vi "Measurement Logic.vi"(8 "error in":errorcluster, 10 "Measurement Context":refnum<class "MeasurementContext.lvclass">, 11 "Measurement Configuration":T2) -> (0 "error out":errorcluster, 2 "Measurement Context out":refnum<class "MeasurementContext.lvclass">, 3 "Measurement Results":T1 {"Load Regulation (mV/mA)" format="%#.5g"})   [LabVIEW 2020, in "LoadRegulation.lvlib"]
uses:
  LoadRegulation.lvlib
  Measurement Configuration.ctl
  Measurement Results.ctl
  RPC Service/MeasurementContext/MeasurementContext.lvclass
  TestInputs.ctl
  Reusables/Advanced Settings.ctl
  Reusables/Prepare Fn Configurations.ctl
  Reusables/Load Output Function.ctl
  Reusables/Stimulus And Measure.ctl
  TestResults.ctl
  e7ccc9a1-0b5d-4153-a5a6-c1ed66e62fb2.vi
panel:
  out "Load Regulation":cluster{"Iload (mA)":dbl[], "Vout (V)":dbl[]}(graph)
  out "Load Regulation (%)":dbl format="%#.3g"
  out "Load Regulation (mV/mA)":dbl format="%#.3g"
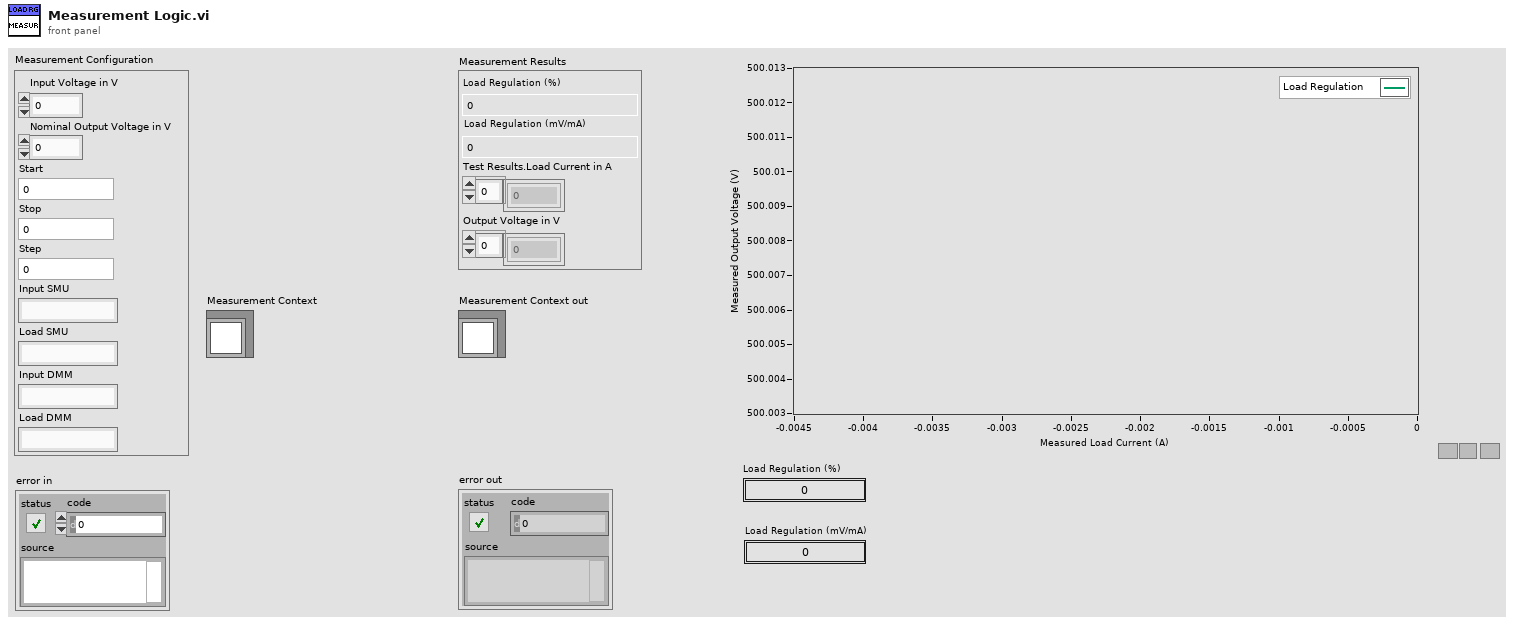
[diagram p1: front panel]
types:
  T1 = typedef "LoadRegulation.lvlib/Measurement Results.ctl" = cluster{"Load Regulation (%)":dbl, "Load Regulation (mV/mA)":dbl, "Test Results.Load Current in A":dbl[], "Output Voltage in V":dbl[]}
  T2 = typedef "LoadRegulation.lvlib/Measurement Configuration.ctl" = cluster{"Input Voltage in V":dbl, "Nominal Output Voltage in V":dbl, "Start":dbl, "Stop":dbl, "Step":dbl, "Input SMU":string, "Load SMU":string, "Input DMM":string, "Load DMM":string}
  T3 = typedef "LoadRegulation.lvlib/TestInputs.ctl" = cluster{"Input Voltage in V":dbl, "Load Current in A":dbl[], "Nominal Output Voltage in V":dbl, "Advance Setting":T4}
  T4 = typedef "Advanced Settings.ctl" = cluster{"Prepare":T5, "Stimulus And Measure":T7}
  T5 = typedef "Prepare Fn Configurations.ctl" = cluster{"Load SMU Output Function":T6}
  T6 = typedef "Load Output Function.ctl" = enum16{"VoltageSource", "CurrentSource"}
  T7 = typedef "Stimulus And Measure.ctl" = cluster{"Loop Delay in milliSecond":u32}
  T8 = typedef "LoadRegulation.lvlib/TestResults.ctl" = cluster{"Input Voltage in V":dbl[], "Input Current in A":dbl[], "Output Voltage in V":dbl[], "Load Current in A":dbl[], "Load Regulation in mV/mA":dbl, "Load Regulation in %":dbl}
  T9 = cluster{"Test Inputs":T3, "Test Results":T8, "Test Results[][]":string[][], "Input SMU":refnum<k15>, "Input DMM":refnum<k15>, "Load DMM":refnum<k15>, "Load SMU":refnum<k15>}
  T10 = cluster{"Load Current in A":dbl[], "Output Voltage in V":dbl[]}
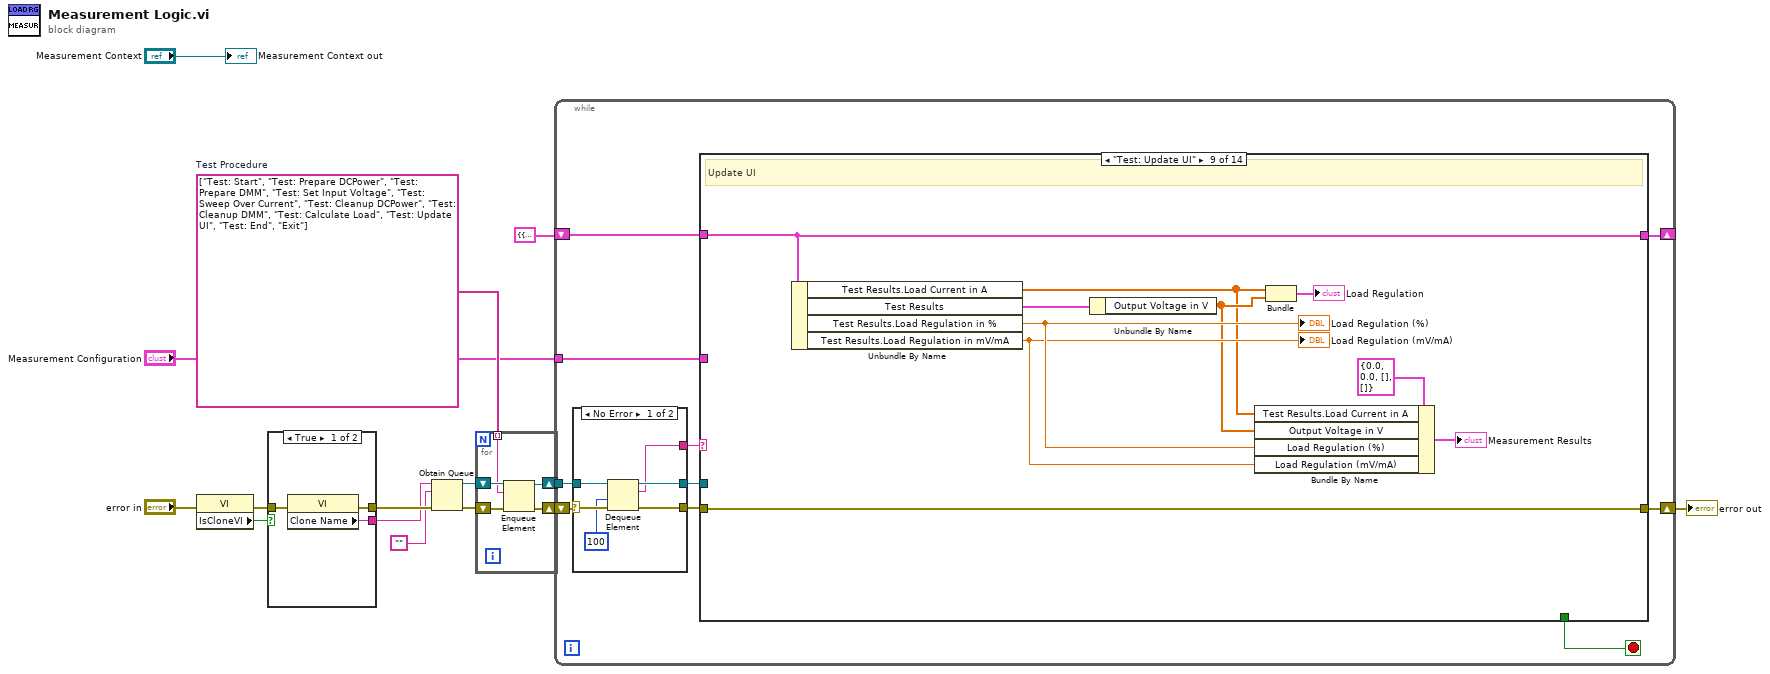
[diagram p0: block diagram]
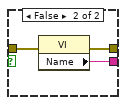
[diagram p2: hidden frame]
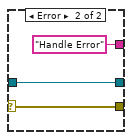
[diagram p3: hidden frame]
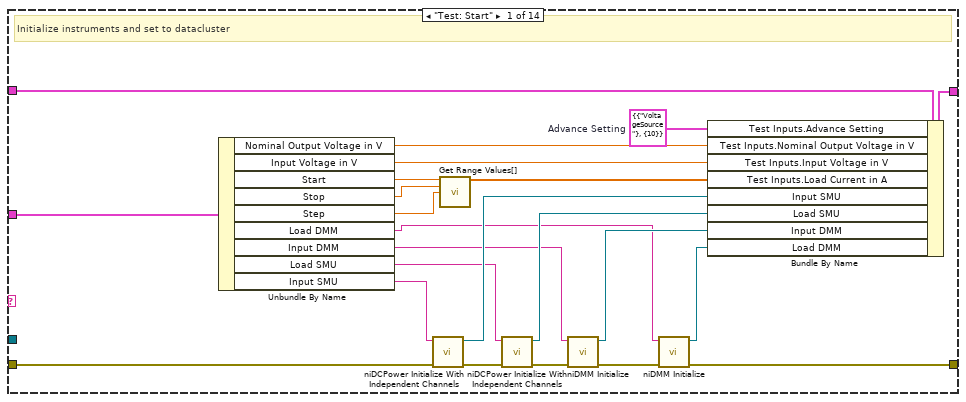
[diagram p4: hidden frame]
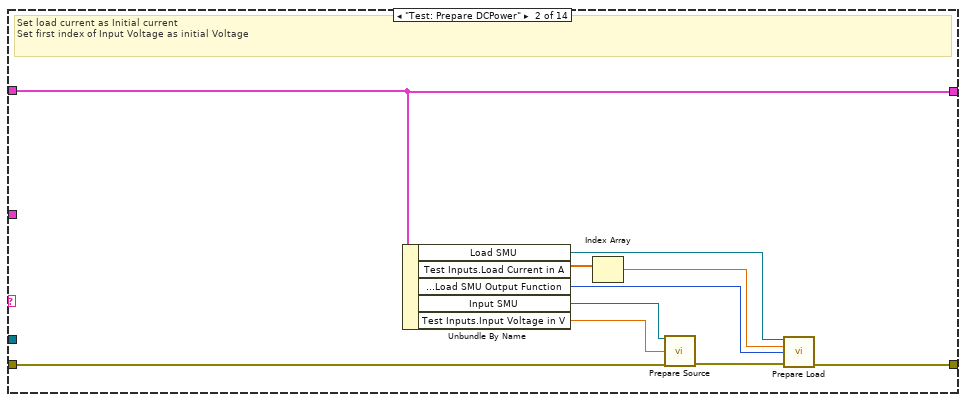
[diagram p5: hidden frame]
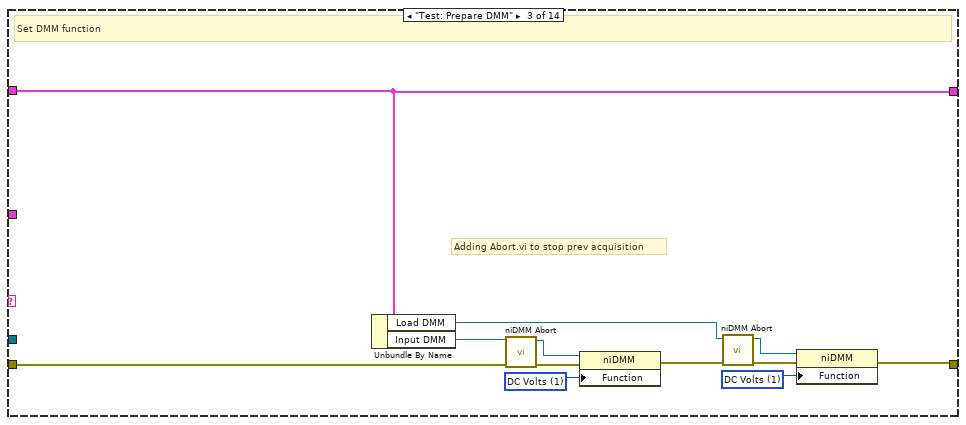
[diagram p6: hidden frame]
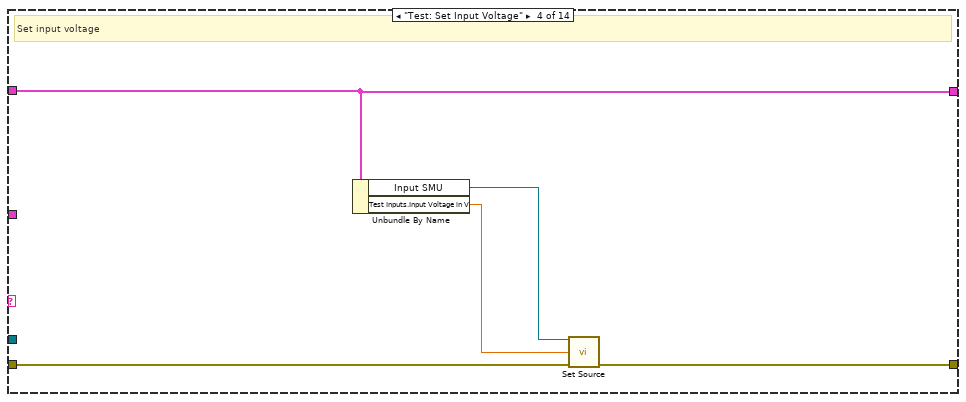
[diagram p7: hidden frame]
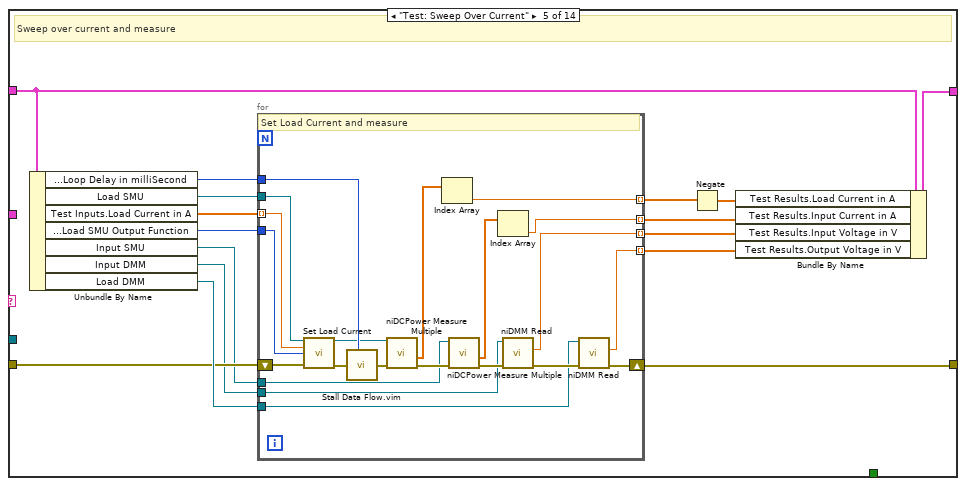
[diagram p8: hidden frame]
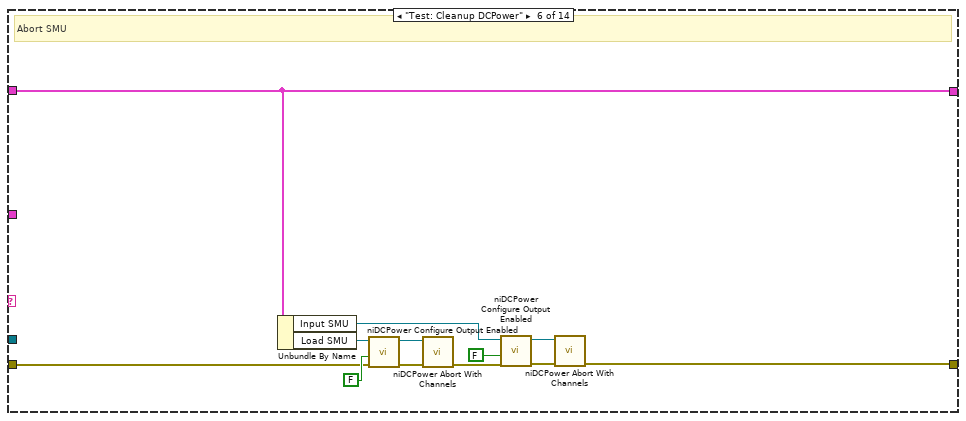
[diagram p9: hidden frame]
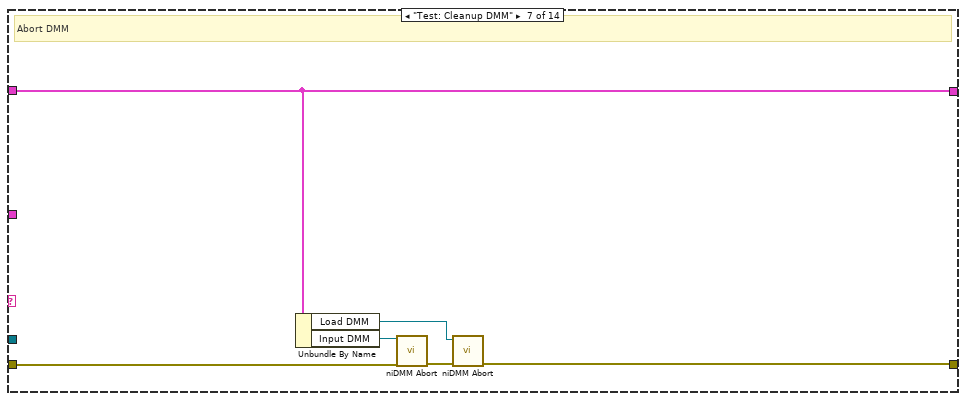
[diagram p10: hidden frame]
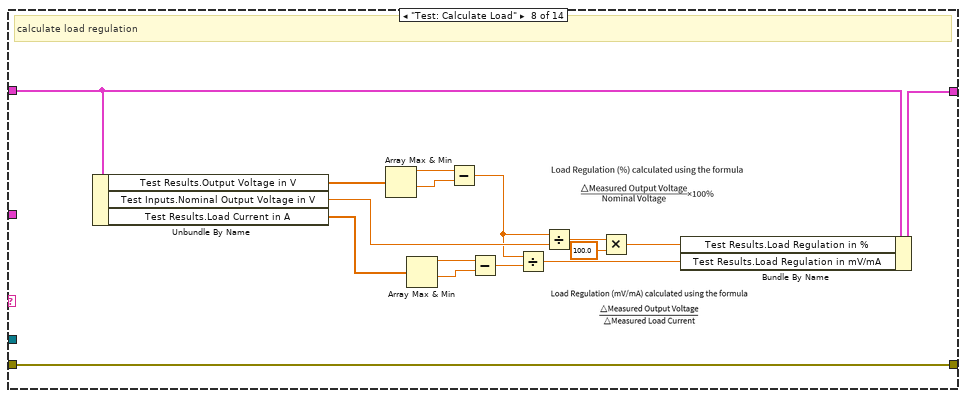
[diagram p11: hidden frame]
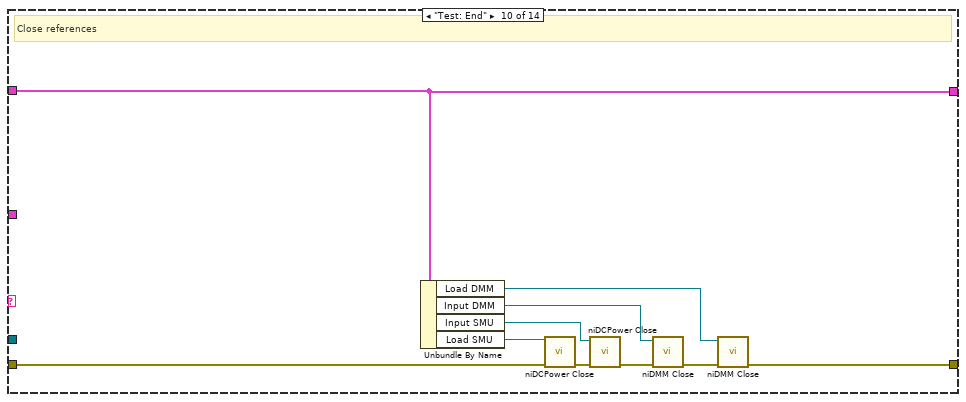
[diagram p12: hidden frame]
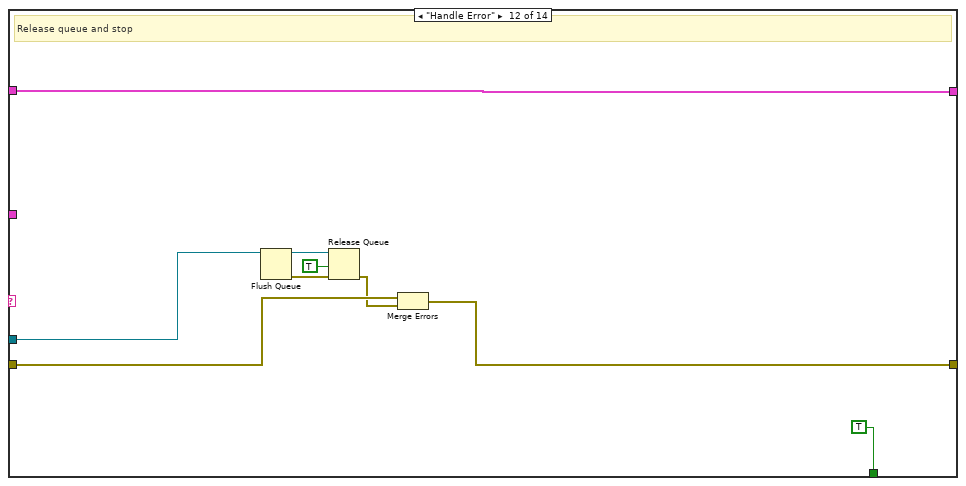
[diagram p14: hidden frame]
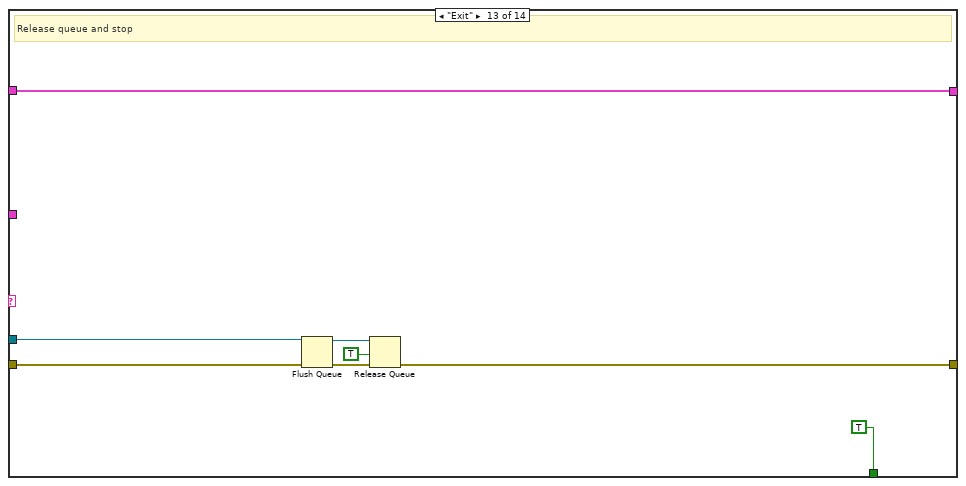
[diagram p15: hidden frame]
diagram:
  w5 = string[] ["Test: Start", "Test: Prepare DCPower", "Test: Prepare DMM", "Test: Set Input Voltage", "Test: Sweep Over Current", "Test: Cleanup DCPower", "Test: Cleanup DMM", "Test: Calculate Load", "Test: Update UI", "Test: End", "Exit"]  # Test Procedure
  n1 = property class="VI"(error in="error in") -> (error out=w8:errorcluster, "IsCloneVI"=w9:bool)  [unwired: 1 in, 1 out]
  n2 = case shown="True" w9 {
    tunnel: [w18 w21] -> w14
    tunnel: [w17 w20] -> w13
    tunnel: w8 -> [w16 w19]
    frame True {
      n3 = property class="VI"(error in=w16) -> (error out=w18:errorcluster, "Clone Name"=w17:string)  [unwired: 1 in, 1 out]
    }
    frame False {
      n4 = property class="VI"(error in=w19) -> (error out=w21:errorcluster, "Name"=w20:string)  [unwired: 1 in, 1 out]
    }
  }
  n5 = Obtain Queue(name (unnamed)=w13, element data type="", error in (no error)=w14) -> (queue out=w11:refnum<queue>, error out=w12:errorcluster)  [unwired: 2 in, 1 out]
  n6 = for {
    shift-right: [w23] -> w6
    shift-left: w12 -> [w26]
    shift-right: [w24] -> w7
    shift-left: w11 -> [w25]
    tunnel: w5 -> [w22] mode=indexing
    n7 = Enqueue Element(queue=w25, element=w22, error in (no error)=w26) -> (queue out=w24:refnum<queue>, error out=w23:errorcluster)  [unwired: 1 in, 1 out]
  }
  n8 = while {
    tunnel: w7 -> [w31]
    shift-right: [w36] -> w3
    shift-left: w6 -> [w32]
    shift-right: [w34] -> _
    shift-left: T9 {"Test Inputs"={"Input Voltage in V"=0.0, "Load Current in A"=[], "Nominal Output Voltage in V"=0.0, "Advance Setting"={"Prepare"={"Load SMU Output Function"=enum."VoltageSource"}, "Stimulus And Measure"={"Loop Delay in milliSecond"=1}}}, "Test Results"={"Input Voltage in V"=[], "Input Current in A"=[], "Output Voltage in V"=[], "Load Current in A"=[], "Load Regulation in mV/mA"=0.0, "Load Regulation in %"=0.0}, "Test Results[][]"=[], "Input SMU"="", "Input DMM"="", "Load DMM"="", "Load SMU"=""} -> [w35]
    tunnel: "Measurement Configuration" -> [w27]
    stop <- w33 stop-if-true
    n9 = case shown="No Error" w32 {
      selector: w32 -> [w42 w45]
      tunnel: [w41 w45] -> w28
      tunnel: w31 -> [w40 w44]
      tunnel: [w39 w44] -> w29
      tunnel: [w38 "Handle Error"] -> w30
      frame No Error {
        n10 = Dequeue Element(queue=w40, timeout in ms (-1)=100, error in (no error)=w42) -> (queue out=w39:refnum<queue>, element=w38:string, error out=w41:errorcluster)  [unwired: 1 out]
      }
      frame Error {
      }
    }
    n11 = case shown="\"Test: Update UI\"" w30 {
      tunnel: w29 -> [_ _ _ _ _ _ _ _ _ _ _ w189 w198 _]
      tunnel: w28 -> [w50 w71 w79 w91 w100 w133 w145 w151 w169 w177 w188 w195 w200 w206]
      tunnel: [w63 w72 w81 w92 w103 w141 w148 w151 w169 w180 w188 w196 w199 w206] -> w36
      tunnel: w35 -> [w67 w77 w87 w95 w101 w140 w150 w152 w174 w186 w187 w197 w205 w207]
      tunnel: [w68 w77 w87 w95 w102 w140 w150 w153 w174 w186 w187 w197 w205 w207] -> w34
      tunnel: [_ _ _ _ _ _ _ _ _ _ _ TRUE TRUE _] -> w33
      tunnel: w27 -> [w46 _ _ _ _ _ _ _ _ _ _ _ _ _]
      frame "Test: Start" {
        w49 = T4 {"Prepare"={"Load SMU Output Function"=enum."VoltageSource"}, "Stimulus And Measure"={"Loop Delay in milliSecond"=10}}  # Advance Setting
        # "Initialize instruments and set to datacluster"
        n12 = Unbundle By Name(w46) -> ("Nominal Output Voltage in V"=w58:dbl, "Input Voltage in V"=w47:dbl, "Start"=w57:dbl, "Stop"=w56:dbl, "Step"=w55:dbl, "Load DMM"=w51:string, "Input DMM"=w52:string, "Load SMU"=w53:string, "Input SMU"=w54:string)
        n13 = call <instrlib>:"niDCPower Initialize With Independent Channels.vi"("error in (no error)"=w50, "resource name"=w54) -> ("error out"=w62:errorcluster, "instrument handle out"=w66:refnum<k15>)  [unwired: 8 in]
        n14 = call "Get Range Values[].vi"("Start"=w57, "Stop"=w56, "Step Size"=w55) -> ("Values[]"=w48:dbl[])  [unwired: 12 in]
        n15 = call <instrlib>:"niDCPower Initialize With Independent Channels.vi"("error in (no error)"=w62, "resource name"=w53) -> ("error out"=w61:errorcluster, "instrument handle out"=w59:refnum<k15>)  [unwired: 8 in]
        n16 = call <instrlib>:"niDMM Initialize.vi"("error in (no error)"=w61, "Instrument Descriptor"=w52) -> ("error out"=w64:errorcluster, "instrument handle out"=w60:refnum<k15>)  [unwired: 8 in]
        n17 = call <instrlib>:"niDMM Initialize.vi"("error in (no error)"=w64, "Instrument Descriptor"=w51) -> ("error out"=w63:errorcluster, "instrument handle out"=w65:refnum<k15>)  [unwired: 8 in]
        n18 = Bundle By Name(cluster=w67, "Test Inputs.Advance Setting"=w49, "Test Inputs.Nominal Output Voltage in V"=w58, "Test Inputs.Input Voltage in V"=w47, "Test Inputs.Load Current in A"=w48, "Input SMU"=w66, "Load SMU"=w59, "Input DMM"=w60, "Load DMM"=w65) -> (w68:T9)
      }
      frame "Test: Prepare DCPower" {
        # "Set load current as Initial current\nSet first index of Input Voltage as initial Voltage"
        n19 = Unbundle By Name(w77) -> ("Load SMU"=w75:refnum<k15>, "Test Inputs.Load Current in A"=w74:dbl[], "Test Inputs.Advance Setting.Prepare.Load SMU Output Function"=w69:T6, "Input SMU"=w76:refnum<k15>, "Test Inputs.Input Voltage in V"=w78:dbl)
        n20 = Index Array(array=w74) -> (element=w70:dbl)  [unwired: 1 in]
        n21 = call "Prepare Source.vi"("instrument handle"=w76, "Initial Voltage Level (V)"=w78, "error in (no error)"=w71) -> ("error out"=w73:errorcluster)  [unwired: 12 in]
        n22 = call "Prepare Load.vi"("instrument handle"=w75, "Load Current Level (A)"=w70, "Load Output Function"=w69, "error in (no error)"=w73) -> ("error out"=w72:errorcluster)  [unwired: 11 in]
      }
      frame "Test: Prepare DMM" {
        w83 = 1 items=["DC Volts"=1, "AC Volts"=2, "DC Current"=3, "AC Current"=4, "2-Wire Resistance"=5, "4-Wire Resistance"=101, "Frequency"=104, "Period"=105, "AC Volts DC Coupled"=1001, "Diode"=1002, "Waveform Voltage"=1003, "Waveform Current"=1004, "Capacitance"=1005, "Inductance"=1006, "Temperature"=108] ("Configuration:Function")
        w90 = 1 items=["DC Volts"=1, "AC Volts"=2, "DC Current"=3, "AC Current"=4, "2-Wire Resistance"=5, "4-Wire Resistance"=101, "Frequency"=104, "Period"=105, "AC Volts DC Coupled"=1001, "Diode"=1002, "Waveform Voltage"=1003, "Waveform Current"=1004, "Capacitance"=1005, "Inductance"=1006, "Temperature"=108] ("Configuration:Function")
        # "Adding Abort.vi to stop prev acquisition"
        # "Set DMM function"
        n23 = Unbundle By Name(w87) -> ("Load DMM"=w80:refnum<k15>, "Input DMM"=w86:refnum<k15>)
        n24 = call <instrlib>:"niDMM Abort.vi"("error in (no error)"=w79, "instrument handle"=w86) -> ("error out"=w89:errorcluster, "instrument handle out"=w88:refnum<k15>)  [unwired: 8 in]
        n25 = property class="niDMM"(reference=w88, error in=w89, "Function"=w90) -> (error out=w82:errorcluster)  [unwired: 1 out]
        n26 = call <instrlib>:"niDMM Abort.vi"("error in (no error)"=w82, "instrument handle"=w80) -> ("error out"=w84:errorcluster, "instrument handle out"=w85:refnum<k15>)  [unwired: 8 in]
        n27 = property class="niDMM"(reference=w85, error in=w84, "Function"=w83) -> (error out=w81:errorcluster)  [unwired: 1 out]
      }
      frame "Test: Set Input Voltage" {
        # "Set input voltage"
        n28 = Unbundle By Name(w95) -> ("Input SMU"=w94:refnum<k15>, "Test Inputs.Input Voltage in V"=w93:dbl)
        n29 = call "Set Source.vi"("instrument handle in"=w94, "Vin in V"=w93, "error in (no error)"=w91) -> ("error out"=w92:errorcluster)  [unwired: 11 in, 1 out]
      }
      frame "Test: Sweep Over Current" {
        # "Sweep over current and measure"
        n30 = Unbundle By Name(w101) -> ("Test Inputs.Advance Setting.Stimulus And Measure.Loop Delay in milliSecond"=w109:u32, "Load SMU"=w111:refnum<k15>, "Test Inputs.Load Current in A"=w110:dbl[], "Test Inputs.Advance Setting.Prepare.Load SMU Output Function"=w99:T6, "Input SMU"=w96:refnum<k15>, "Input DMM"=w97:refnum<k15>, "Load DMM"=w108:refnum<k15>)
        n31 = for {
          tunnel: w111 -> [w131]
          tunnel: w110 -> [w114] mode=indexing
          tunnel: w109 -> [w129]
          tunnel: w97 -> [w122]
          tunnel: w108 -> [w121]
          tunnel: [w115] -> w107 mode=indexing
          tunnel: [w116] -> w106 mode=indexing
          tunnel: [w120] -> w105 mode=indexing
          tunnel: [w119] -> w104 mode=indexing
          shift-right: [w118] -> w103
          shift-left: w100 -> [w132]
          tunnel: w99 -> [w113]
          tunnel: w96 -> [w112]
          # "Set Load Current and measure"
          n32 = call "Set Load Current.vi"("instrument handle in"=w131, "current level"=w114, "OutputFunction"=w113, "error in (no error)"=w132) -> ("instrument handle out"=w117:refnum<k15>, "error out"=w130:errorcluster)  [unwired: 10 in]
          n33 = call "Stall Data Flow.vim"("value in"=w130, "milliseconds to wait"=w129) -> ("value out"=w123:errorcluster)  [unwired: 1 out]
          n34 = call <instrlib>:"niDCPower Measure Multiple.vi"("error in (no error)"=w123, "instrument handle"=w117) -> ("error out"=w125:errorcluster, "current measurements"=w128:dbl[])  [unwired: 6 in, 2 out]
          n35 = Index Array(array=w128) -> (element=w116:dbl)  [unwired: 1 in]
          n36 = call <instrlib>:"niDCPower Measure Multiple.vi"("error in (no error)"=w125, "instrument handle"=w112) -> ("error out"=w124:errorcluster, "current measurements"=w126:dbl[])  [unwired: 6 in, 2 out]
          n37 = Index Array(array=w126) -> (element=w115:dbl)  [unwired: 1 in]
          n38 = call <instrlib>:"niDMM Read.vi"("error in (no error)"=w124, "instrument handle"=w122) -> ("error out"=w127:errorcluster, "Measurement"=w120:dbl)  [unwired: 7 in, 1 out]
          n39 = call <instrlib>:"niDMM Read.vi"("error in (no error)"=w127, "instrument handle"=w121) -> ("error out"=w118:errorcluster, "Measurement"=w119:dbl)  [unwired: 7 in, 1 out]
        }
        n40 = Negate(x=w106) -> (-x=w98:dbl[])
        n41 = Bundle By Name(cluster=w101, "Test Results.Load Current in A"=w98, "Test Results.Input Current in A"=w107, "Test Results.Input Voltage in V"=w105, "Test Results.Output Voltage in V"=w104) -> (w102:T9)
      }
      frame "Test: Cleanup DCPower" {
        # "Abort SMU"
        n42 = Unbundle By Name(w140) -> ("Input SMU"=w139:refnum<k15>, "Load SMU"=w134:refnum<k15>)
        n43 = call <instrlib>:"niDCPower Configure Output Enabled.vi"("error in (no error)"=w133, "output enabled"=FALSE, "instrument handle"=w134) -> ("error out"=w135:errorcluster, "instrument handle out"=w138:refnum<k15>)  [unwired: 7 in]
        n44 = call <instrlib>:"niDCPower Abort With Channels.vi"("error in (no error)"=w135, "instrument handle"=w138) -> ("error out"=w136:errorcluster)  [unwired: 8 in, 1 out]
        n45 = call <instrlib>:"niDCPower Configure Output Enabled.vi"("error in (no error)"=w136, "output enabled"=FALSE, "instrument handle"=w139) -> ("error out"=w143:errorcluster, "instrument handle out"=w142:refnum<k15>)  [unwired: 7 in]
        n46 = call <instrlib>:"niDCPower Abort With Channels.vi"("error in (no error)"=w143, "instrument handle"=w142) -> ("error out"=w141:errorcluster)  [unwired: 8 in, 1 out]
      }
      frame "Test: Cleanup DMM" {
        # "Abort DMM"
        n47 = Unbundle By Name(w150) -> ("Load DMM"=w147:refnum<k15>, "Input DMM"=w146:refnum<k15>)
        n48 = call <instrlib>:"niDMM Abort.vi"("error in (no error)"=w145, "instrument handle"=w146) -> ("error out"=w149:errorcluster)  [unwired: 8 in, 1 out]
        n49 = call <instrlib>:"niDMM Abort.vi"("error in (no error)"=w149, "instrument handle"=w147) -> ("error out"=w148:errorcluster)  [unwired: 8 in, 1 out]
      }
      frame "Test: Calculate Load" {
        # "calculate load regulation"
        n50 = Unbundle By Name(w152) -> ("Test Results.Output Voltage in V"=w163:dbl[], "Test Inputs.Nominal Output Voltage in V"=w161:dbl, "Test Results.Load Current in A"=w158:dbl[])
        n51 = Array Max & Min(array=w163) -> (max value=w166:dbl, min value=w162:dbl)  [unwired: 2 out]
        n52 = Array Max & Min(array=w158) -> (max value=w159:dbl, min value=w160:dbl)  [unwired: 2 out]
        n53 = Subtract(x=w166, y=w162) -> (x-y=w157:dbl)
        n54 = Subtract(x=w159, y=w160) -> (x-y=w156:dbl)
        n55 = Divide(x=w157, y=w156) -> (x/y=w155:dbl)
        n56 = Divide(x=w157, y=w161) -> (x/y=w165:dbl)
        n57 = Multiply(x=w165, y=100.0) -> (x*y=w164:dbl)
        n58 = Bundle By Name(cluster=w152, "Test Results.Load Regulation in %"=w164, "Test Results.Load Regulation in mV/mA"=w155) -> (w153:T9)
      }
      frame "Test: Update UI" {
        # "Update UI"
        n59 = Unbundle By Name(w174) -> ("Test Results.Load Current in A"=w170:dbl[], "Test Results"=w176:T8, "Test Results.Load Regulation in %"=w173:dbl, "Test Results.Load Regulation in mV/mA"=w172:dbl)
        "Load Regulation (%)" <- w173
        "Load Regulation (mV/mA)" <- w172
        n60 = Unbundle By Name(w176) -> ("Output Voltage in V"=w171:dbl[])
        n61 = Bundle By Name(cluster=T1 {"Load Regulation (%)"=0.0, "Load Regulation (mV/mA)"=0.0, "Test Results.Load Current in A"=[], "Output Voltage in V"=[]} ("Measurement Results"), "Test Results.Load Current in A"=w170, "Output Voltage in V"=w171, "Load Regulation (%)"=w173, "Load Regulation (mV/mA)"=w172) -> (→"Measurement Results":T1)
        n62 = Bundle("Load Current in A"=w170, "Output Voltage in V"=w171) -> (→"Load Regulation":T10)  [unwired: 1 in]
      }
      frame "Test: End" {
        # "Close references"
        n63 = Unbundle By Name(w186) -> ("Load DMM"=w181:refnum<k15>, "Input DMM"=w182:refnum<k15>, "Input SMU"=w185:refnum<k15>, "Load SMU"=w179:refnum<k15>)
        n64 = call <instrlib>:"niDCPower Close.vi"("error in (no error)"=w177, "instrument handle"=w179) -> ("error out"=w178:errorcluster)  [unwired: 9 in]
        n65 = call <instrlib>:"niDCPower Close.vi"("error in (no error)"=w178, "instrument handle"=w185) -> ("error out"=w184:errorcluster)  [unwired: 9 in]
        n66 = call <instrlib>:"niDMM Close.vi"("error in (no error)"=w184, "instrument handle"=w182) -> ("error out"=w183:errorcluster)  [unwired: 9 in]
        n67 = call <instrlib>:"niDMM Close.vi"("error in (no error)"=w183, "instrument handle"=w181) -> ("error out"=w180:errorcluster)  [unwired: 9 in]
      }
      frame "----Misc------" {
      }
      frame "Handle Error" {
        # "Release queue and stop"
        n68 = Flush Queue(queue=w189) -> (queue out=w193:refnum<queue>, error out=w192:errorcluster)  [unwired: 1 in, 1 out]
        n69 = Release Queue(queue=w193, force destroy? (F)=TRUE, error in (no error)=w192) -> (error out=w190:errorcluster)  [unwired: 2 out]
        n70 = Merge Errors(w195, w190) -> (w196:errorcluster)
      }
      frame "Exit" {
        # "Release queue and stop"
        n71 = Flush Queue(queue=w198, error in (no error)=w200) -> (queue out=w203:refnum<queue>, error out=w202:errorcluster)  [unwired: 1 out]
        n72 = Release Queue(queue=w203, force destroy? (F)=TRUE, error in (no error)=w202) -> (error out=w199:errorcluster)  [unwired: 2 out]
      }
      frame "", Default {
        # "Do nothing"
      }
    }
  }
  "error out" <- w3
  "Measurement Context out" <- "Measurement Context"
